vi "ExportOtherFileContent.vi"(6 "CodeSchema":string, 8 "error in (no error)":errorcluster, 10 "ILabVIEWItem in":refnum<class "ILabVIEWItem.lvclass">, 11 "CGrapherDGML in":refnum<class "CGrapherDGML.lvclass">) -> (0 "error out":errorcluster, 1 "Links":T1, 2 "Nodes":T1, 3 "CGrapherDGML":refnum<class "CGrapherDGML.lvclass">)   [LabVIEW 2020, in "DefaultExtensions.lvlib" / "CGrapherDGML.lvclass"]
uses:
  CGrapherDGML.lvclass
  LabVIEWObjectInterfaces/ILabVIEWItem/ILabVIEWItem.lvclass
  LabVIEWItem/CLabVIEWItem/ConnectionSet.ctl
  CGrapherDGML.lvclass/CGrapherDGML.ctl
  LabVIEWItem/CLabVIEWItem/CLabVIEWItem.lvclass
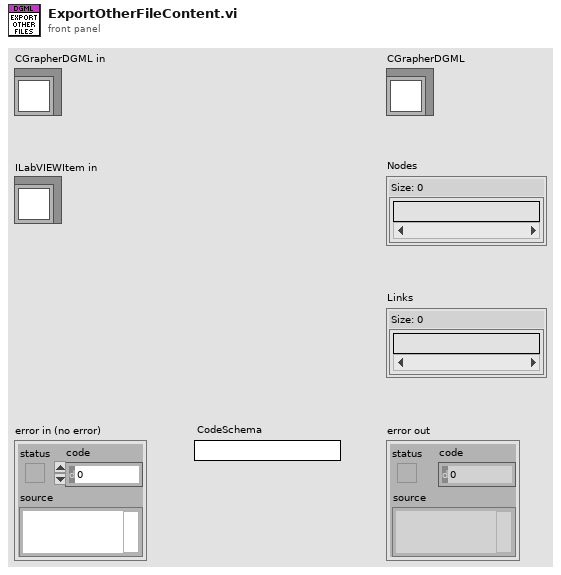
[diagram p1: front panel]
types:
  T1 = typedef "LabVIEWItem.lvlib/CLabVIEWItem.lvclass/ConnectionSet.ctl" = set{string}
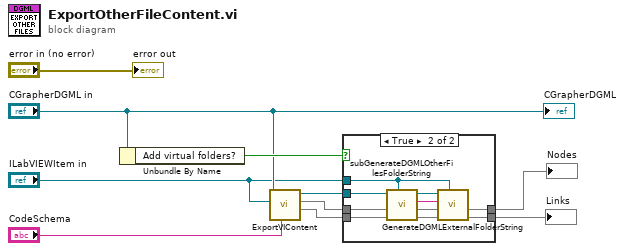
[diagram p0: block diagram]
diagram:
  n1 = Unbundle By Name("CGrapherDGML in") -> ("Add virtual folders?"=w7:bool)
  n2 = call-dynamic "ExportVIContent.vi"("CodeSchema"="CodeSchema", "ILabVIEWItem in"="ILabVIEWItem in", "CGrapherDGML in"="CGrapherDGML in") -> ("Links"=w1:T1, "Nodes"=w2:T1, "CGrapherDGML"=w5:refnum<class "CGrapherDGML.lvclass">)  [unwired: 6 in]
  n3 = case shown="True" w7 {
    tunnel: w1 -> [w11 w14]
    tunnel: [w11 w16] -> w10
    tunnel: w2 -> [w12 w15]
    tunnel: [w12 w17] -> w9
    tunnel: "ILabVIEWItem in" -> [_ w13]
    tunnel: w5 -> [_ w18]
    frame False {
    }
    frame True {
      n4 = call "subGenerateDGMLOtherFilesFolderString.vi"("ILabVIEWItem in"=w13, "Links in"=w14, "Nodes in"=w15, "CGrapherDGML in"=w18) -> ("Links"=w22:T1, "Nodes"=w19:T1, "Path"=w20:string, "CGrapherDGML"=w21:refnum<class "CGrapherDGML.lvclass">)  [unwired: 4 in]
      n5 = call-dynamic "GenerateDGMLExternalFolderString.vi"("ILabVIEWItem in"=w13, "Links in"=w22, "Nodes in"=w19, "Path in"=w20, "CGrapherDGML in"=w21) -> ("Links"=w16:T1, "Nodes"=w17:T1)  [unwired: 4 in, 1 out]
    }
  }
  "Nodes" <- w9
  "Links" <- w10
  "error out" <- "error in (no error)"
  "CGrapherDGML" <- "CGrapherDGML in"
